vi "Write CellStyleWordWrap.vi"(8 "error in (no error)":errorcluster, 10 "CellStyleWordWrap":bool=TRUE, 11 "DataGridView in":refnum<class "DataGridView.lvclass">) -> (0 "error out":errorcluster, 3 "DataGridView out":refnum<class "DataGridView.lvclass">)   [LabVIEW 2014, in "DataGridView.lvclass"]
uses:
  DataGridView.lvclass
  System.Windows.Forms
  DataGridView.lvclass/DataGridView.ctl
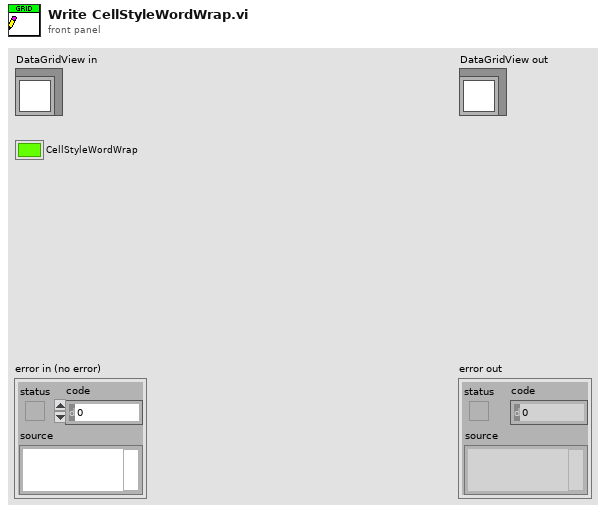
[diagram p1: front panel]
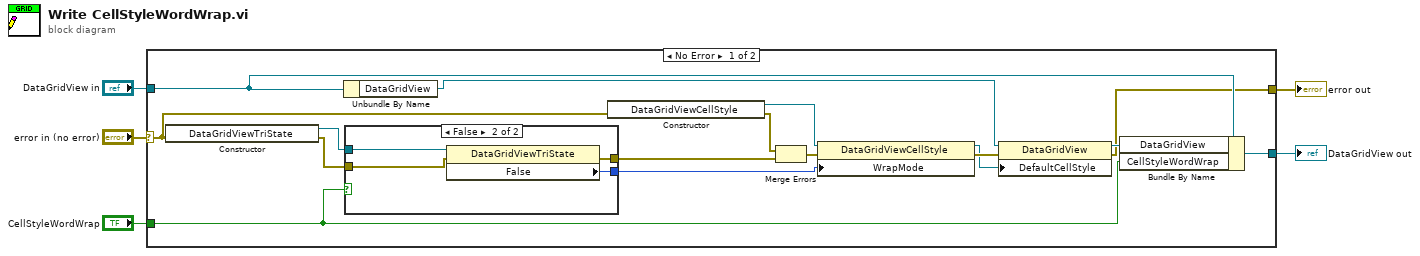
[diagram p0: block diagram]
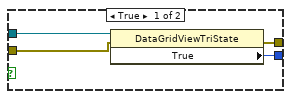
[diagram p2: hidden frame]
diagram:
  n1 = case shown="No Error" "error in (no error)" {
    selector: "error in (no error)" -> [w7 w30]
    tunnel: [w6 w30] -> w4
    tunnel: [w8 w31] -> w2
    tunnel: "DataGridView in" -> [w9 w31]
    tunnel: "CellStyleWordWrap" -> [w10 _]
    frame No Error {
      n2 = constructor class="DataGridViewTriState"(error in=w7) -> (reference out=w19:refnum<k24>, error out=w20:errorcluster)  [unwired: 2 in, 1 out]
      n3 = Unbundle By Name(w9) -> ("DataGridView"=w11:refnum<k24>)
      n4 = case shown="False" w10 {
        tunnel: w20 -> [w25 w29]
        tunnel: w19 -> [w24 w28]
        tunnel: [w23 w27] -> w18
        tunnel: [w22 w26] -> w16
        frame True {
          n5 = property class="DataGridViewTriState"(reference=w24, error in=w25) -> (error out=w22:errorcluster, "True"=w23:i32)  [unwired: 1 out]
        }
        frame False {
          n6 = property class="DataGridViewTriState"(reference=w28, error in=w29) -> (error out=w26:errorcluster, "False"=w27:i32)  [unwired: 1 out]
        }
      }
      n7 = constructor class="DataGridViewCellStyle"(error in=w7) -> (reference out=w15:refnum<k24>, error out=w12:errorcluster)  [unwired: 2 in, 1 out]
      n8 = Merge Errors(w12, w16) -> (w13:errorcluster)
      n9 = property class="DataGridViewCellStyle"(reference=w15, error in=w13, "WrapMode"=w18) -> (reference out=w14:refnum<k24>, error out=w17:errorcluster)
      n10 = property class="DataGridView"(reference=w11, error in=w17, "DefaultCellStyle"=w14) -> (reference out=w21:refnum<k24>, error out=w6:errorcluster)
      n11 = Bundle By Name(cluster=w9, "DataGridView"=w21, "CellStyleWordWrap"=w10) -> (w8:refnum<class "DataGridView.lvclass">)
    }
    frame Error {
    }
  }
  "error out" <- w4
  "DataGridView out" <- w2
